vi "Engine Initialize.vi"(8 "error in (no error)":errorcluster, 11 "Paramters":variant) -> (0 "error out":errorcluster, 1 "CD Out Buffer":dbl[](array[numeric]), 2 "CD In Buffer":dbl[](array[numeric]), 3 "Engine Run Time Data":T1)   [LabVIEW 2017]
uses:
  Controls/Channel Mode.ctl
  NI 272x Resistive Simulation Custom Device Shared.lvlib
  <instrlib>/ni272xReferenceVIs/ni272xReferenceVIs.llb/ni272x Callendar-Van Dusen RTD Parameters.ctl
  Controls/Compiled HW Channel.ctl
  Controls/Compiled Connect Channel.ctl
  Controls/Compiled Engine Data.ctl
  Controls/Engine Run Time Data.ctl
  NI 272x Resistive Simulation Custom Device Engine.lvlib
  <instrlib>/ni272xReferenceVIs/ni272xReferenceVIs.llb/ni272x Reference.ctl
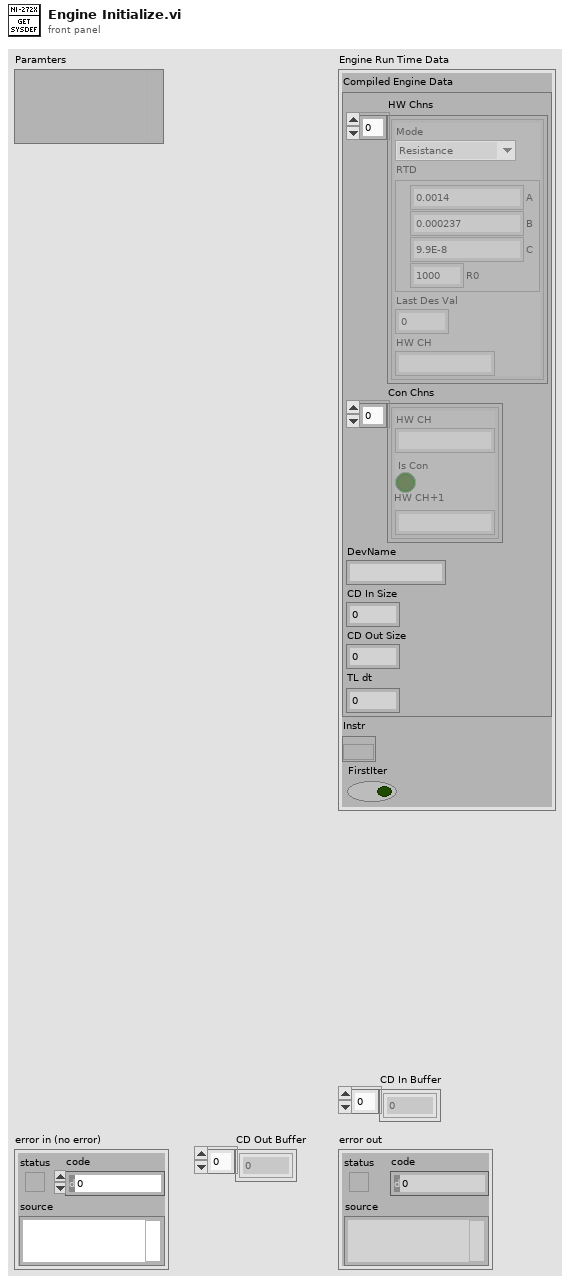
[diagram p1: front panel]
types:
  T1 = typedef "NI 272x Resistive Simulation Custom Device Engine.lvlib/Engine Run Time Data.ctl" = cluster{"Compiled Engine Data":T2, "Instr":T7, "FirstIter":bool}
  T2 = typedef "NI 272x Resistive Simulation Custom Device Shared.lvlib/Compiled Engine Data.ctl" = cluster{"HW Chns":T3[], "Con Chns":T6[], "DevName":string, "CD In Size":i32, "CD Out Size":i32, "TL dt":i64}
  T3 = typedef "NI 272x Resistive Simulation Custom Device Shared.lvlib/Compiled HW Channel.ctl" = cluster{"Mode":T4, "RTD":T5, "Last Des Val":dbl, "HW CH":string}
  T4 = typedef "NI 272x Resistive Simulation Custom Device Shared.lvlib/Channel Mode.ctl" = enum16{"Resistance", "RTD Temperature"}
  T5 = typedef "ni272x Callendar-Van Dusen RTD Parameters.ctl" = cluster{"A":dbl, "B":dbl, "C":dbl, "R0":dbl}
  T6 = typedef "NI 272x Resistive Simulation Custom Device Shared.lvlib/Compiled Connect Channel.ctl" = cluster{"HW CH":string, "Is Con":bool, "HW CH+1":string}
  T7 = typedef "ni272x Reference.ctl" = refnum<k20>
  T8 = typedef "NI 272x Resistive Simulation Custom Device Engine.lvlib/Engine Run Time Data.ctl" = cluster{"Compiled Engine Data":T9, "Instr":T7, "FirstIter":bool}
  T9 = typedef "NI 272x Resistive Simulation Custom Device Shared.lvlib/Compiled Engine Data.ctl" = cluster{"HW Chns":T3[], "Con Chns":T6[], "DevName":string, "TL dt":i64}
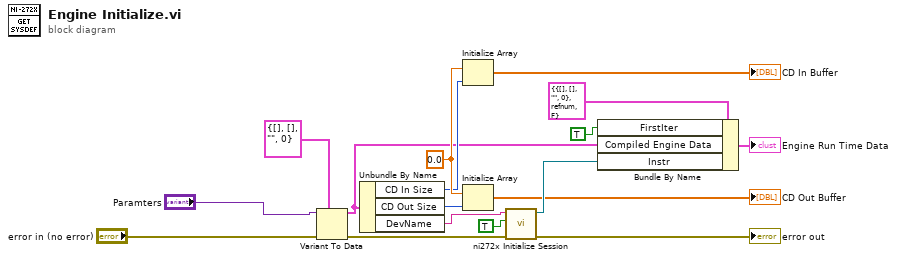
[diagram p0: block diagram]
diagram:
  w14 = 0.0 ("element")
  n1 = Variant To Data(error in="error in (no error)", type=T9 {"HW Chns"=[], "Con Chns"=[], "DevName"="", "TL dt"=0} ("Compiled Engine Data"), Variant="Paramters") -> (data=w11:T9, error out=w9:errorcluster)
  n2 = Unbundle By Name(w11) -> ("CD In Size"=w13:i32, "CD Out Size"=w12:i32, "DevName"=w8:string)
  n3 = Initialize Array(w14, w13) -> (→"CD In Buffer":dbl[])
  n4 = Initialize Array(w14, w12) -> (→"CD Out Buffer":dbl[])
  n5 = call <instrlib>:"ni272x Initialize Session.vi"("error in (no error)"=w9, "reset device (T)"=TRUE, "DAQmx Device Name"=w8) -> ("error out"=→"error out":errorcluster, "instrument handle out"=w5:T7)  [unwired: 7 out]
  n6 = Bundle By Name(cluster=T8 {"Compiled Engine Data"={"HW Chns"=[], "Con Chns"=[], "DevName"="", "TL dt"=0}, "Instr"=refnum, "FirstIter"=FALSE} ("Engine Run Time Data"), "FirstIter"=TRUE, "Compiled Engine Data"=w11, "Instr"=w5) -> (→"Engine Run Time Data":T8)
